vi "go to position.vi"(6 "wait for reply (T)":bool=TRUE, 7 "Pause Time [ms]":i32=50, 8 "error in":errorcluster, 9 "Velocity [rpm]":i32=5, 10 "Position":dbl, 11 "Module ID":i32=-1) -> (0 "error out":errorcluster, 1 "timed out?":bool, 2 "Position 2":dbl)   [LabVIEW 2025, in "Motor.lvlib"]
doc: "_____\nCreated using DQMH Framework: Event Scripter 7.1.2.1547."
uses:
  Motor.lvlib
  go to position Argument--cluster.ctl
  go to position (Reply Payload)--cluster.ctl
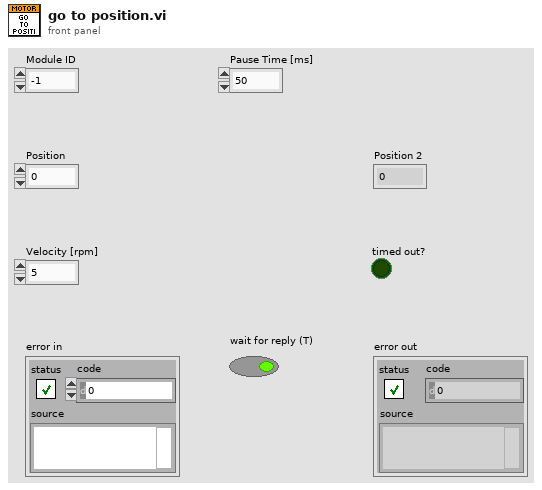
[diagram p1: front panel]
types:
  T1 = typedef "Motor.lvlib/go to position Argument--cluster.ctl" = cluster{"Module ID":i32, "Position":dbl, "Velocity [rpm]":i32, "Pause Time [ms]":i32, "Wait Notifier":refnum<notifier>, "wait for reply":bool}
  T2 = typedef "Motor.lvlib/Request Events--cluster.ctl" = cluster{"Stop Module":refnum<user-event>, "Show Panel":refnum<user-event>, "Hide Panel":refnum<user-event>, "Show Diagram":refnum<user-event>, "Get Module Execution Status":refnum<user-event>, "close":refnum<user-event>, "init":refnum<user-event>, "clear error":refnum<user-event>, "read config":refnum<user-event>, "read position":refnum<user-event>, "go to position":refnum<user-event>}
  T3 = typedef "Motor.lvlib/go to position (Reply Payload)--cluster.ctl" = cluster{"Module ID":i32, "Position":dbl, "error":errorcluster}
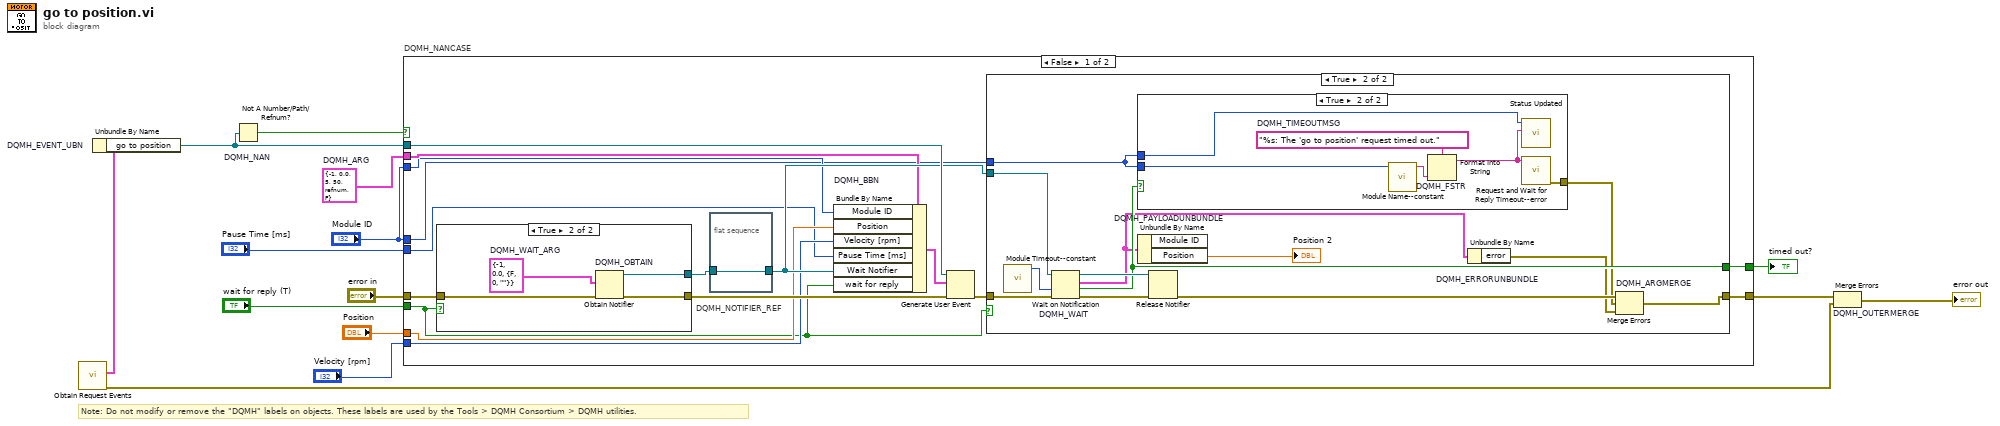
[diagram p0: block diagram]
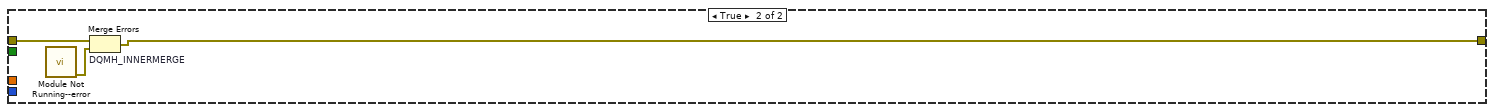
[diagram p5: hidden frame]
diagram:
  w8 = T1 {"Module ID"=-1, "Position"=0.0, "Velocity [rpm]"=5, "Pause Time [ms]"=50, "Wait Notifier"=refnum, "wait for reply"=FALSE}  # DQMH_ARG
  # "Note: Do not modify or remove the \"DQMH\" labels on objects. These labels are used by the Tools > DQMH Consortium > DQMH utilities."
  n1 = call "Obtain Request Events.vi"() -> ("error out"=w2:errorcluster, "Motor Request Events"=w1:T2)  [unwired: 10 in]
  n2 = Unbundle By Name "DQMH_EVENT_UBN"(w1) -> ("go to position"=w12:refnum<user-event>)
  n3 = Not A Number/Path/Refnum? "DQMH_NAN"(number/path/refnum=w12) -> (NaN/Path/Refnum?=w11:bool)
  n4 = case "DQMH_NANCASE" shown="False" w11 {
    tunnel: "error in" -> [w30 w59]
    tunnel: w12 -> [w28 _]
    tunnel: [w25 w58] -> w9
    tunnel: [w26 _] -> w10
    tunnel: w8 -> [w21 _]
    tunnel: "Module ID" -> [w20 _]
    tunnel: "Position" -> [w19 _]
    tunnel: "Velocity [rpm]" -> [w18 _]
    tunnel: "Pause Time [ms]" -> [w17 _]
    tunnel: "Module ID" -> [w16 _]
    tunnel: "wait for reply (T)" -> [w15 _]
    frame False {
      n5 = case shown="True" w15 {
        tunnel: w30 -> [w52 w56]
        tunnel: [w52 w55] -> w27
        tunnel: [_ w53] -> w23
        frame False {
        }
        frame True {
          w54 = T3 {"Module ID"=-1, "Position"=0.0, "error"={"status"=FALSE, "code"=0, "source"=""}}  # DQMH_WAIT_ARG
          n6 = Obtain Notifier "DQMH_OBTAIN"(notification data type=w54, error in (no error)=w56) -> (notifier out=w53:refnum<notifier>, error out=w55:errorcluster)  [unwired: 2 in, 1 out]
        }
      }
      n7 = flat-sequence "DQMH_NOTIFIER_REF" {
        tunnel: w23 -> [w31]
        tunnel: [w31] -> w22
        frame #0 {
        }
      }
      n8 = Bundle By Name "DQMH_BBN"(cluster=w21, "Module ID"=w20, "Position"=w19, "Velocity [rpm]"=w18, "Pause Time [ms]"=w17, "Wait Notifier"=w22, "wait for reply"=w15) -> (w24:T1)
      n9 = Generate User Event(user event=w28, event data cluster=w24, error in=w27) -> (error out=w29:errorcluster)  [unwired: 1 in, 1 out]
      n10 = case shown="True" w15 {
        tunnel: w29 -> [w32 w45]
        tunnel: w22 -> [_ w44]
        tunnel: [_ w42] -> w26
        tunnel: [w32 w41] -> w25
        tunnel: w16 -> [_ w33]
        frame False {
        }
        frame True {
          n11 = call "Module Timeout--constant.vi"() -> ("Module Timeout"=w35:i32)  [unwired: 11 in]
          n12 = Wait on Notification "DQMH_WAIT"(notifier=w44, timeout in ms (-1)=w35, error in (no error)=w45) -> (notifier out=w43:refnum<notifier>, notification=w36:T3, timed out?=w42:bool, error out=w40:errorcluster)  [unwired: 1 in]
          n13 = case shown="True" w42 {
            tunnel: [_ w49] -> w37
            tunnel: w33 -> [_ w47]
            tunnel: w33 -> [_ w46]
            frame False {
            }
            frame True {
              w51 = "%s: The 'go to position' request timed out."  # DQMH_TIMEOUTMSG
              n14 = call "Module Name--constant.vi"("Module ID"=w46) -> ("Module Name"=w48:string)  [unwired: 10 in]
              n15 = Format Into String "DQMH_FSTR"(format string=w51, w48) -> (resulting string=w50:string)  [unwired: 2 in, 1 out]
              n16 = call "Status Updated.vi"("Status"=w50, "Module ID"=w47) -> ()  [unwired: 9 in, 1 out]
              n17 = call "Request and Wait for Reply Timeout--error.vi"("Error Message"=w50) -> ("error out"=w49:errorcluster)  [unwired: 10 in]
            }
          }
          n18 = Unbundle By Name "DQMH_PAYLOADUNBUNDLE"(w36) -> ("Position"=→"Position 2":dbl)  [unwired: 1 out]
          n19 = Release Notifier(notifier=w43, error in (no error)=w40) -> (error out=w39:errorcluster)  [unwired: 1 in, 2 out]
          n20 = Unbundle By Name "DQMH_ERRORUNBUNDLE"(w36) -> ("error"=w38:errorcluster)
          n21 = Merge Errors "DQMH_ARGMERGE"(w39, w37, w38) -> (w41:errorcluster)
        }
      }
    }
    frame True {
      n22 = call "Module Not Running--error.vi"() -> ("error out"=w57:errorcluster)  [unwired: 11 in]
      n23 = Merge Errors "DQMH_INNERMERGE"(w59, w57) -> (w58:errorcluster)
    }
  }
  "timed out?" <- w10
  n24 = Merge Errors "DQMH_OUTERMERGE"(w9, w2) -> (→"error out":errorcluster)
